vi "Open File.vi"(8 "error in (no error)":errorcluster, 11 "Macro in":refnum<class "Macro.lvclass">) -> (0 "error out":errorcluster, 3 "Macro out":refnum<class "Macro.lvclass">)   [LabVIEW 2020, in "MacroAssert.lvlib" / "Macro.lvclass"]
uses:
  Macro.lvclass
  <vilib>/Utility/config.llb/NI_LVConfig.lvlib
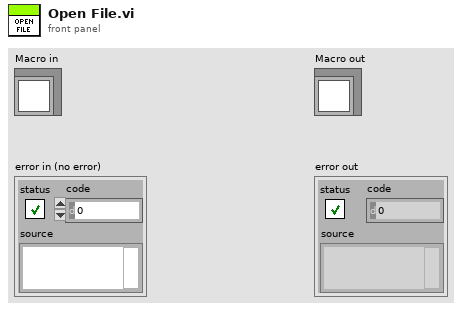
[diagram p1: front panel]
types:
  T1 = typedef "NI_LVConfig.lvlib/Config Data RefNum.ctl" = refnum<k1>
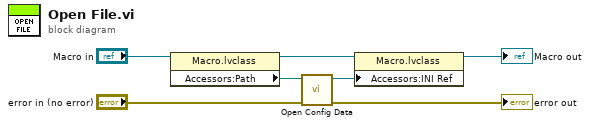
[diagram p0: block diagram]
diagram:
  n1 = property class="Macro.lvclass"(reference="Macro in") -> (reference out=w6:refnum<class "Macro.lvclass">, "Accessors:Path"=w7:path)  [unwired: 1 in, 1 out]
  n2 = call <vilib>:"Open Config Data.vi"("error in (no error)"="error in (no error)", "configuration file path"=w7) -> ("error out"=→"error out":errorcluster, "refnum"=w5:T1)  [unwired: 7 in, 1 out]
  n3 = property class="Macro.lvclass"(reference=w6, "Accessors:INI Ref"=w5) -> (reference out=→"Macro out":refnum<class "Macro.lvclass">)  [unwired: 1 in, 1 out]
